vi "_Recursively Set BD Cluster Autosizing Property.vi"(8 "error in (no error)":errorcluster, 10 "type":T1(ring), 11 "SelList[]":refnum<vi>[](array[refnum])) -> (0 "error out":errorcluster, 3 "changed?":bool)   [LabVIEW 2017, in "Cluster AutoSizing.lvlib"]
uses:
  Cluster AutoSizing.lvlib
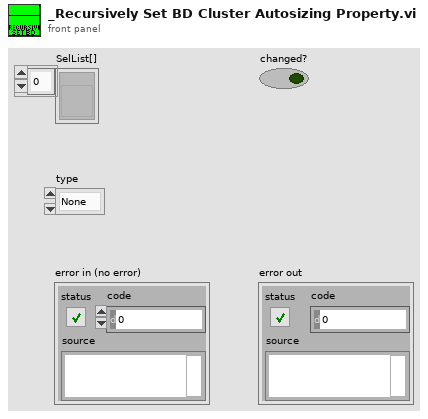
[diagram p1: front panel]
types:
  T1 = enum16{"None", "Size to Fit", "Arrange Horizontally", "Arrange Veritcally"}
  T2 = enum32{"None", "Size to Fit", "Arrange Horizontally", "Arrange Vertically"}
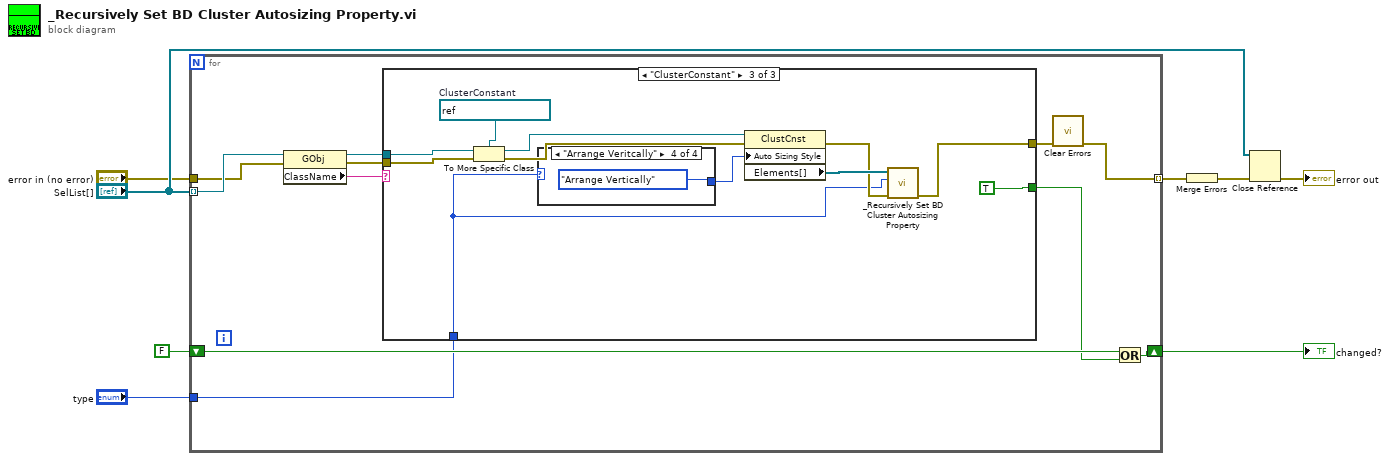
[diagram p0: block diagram]
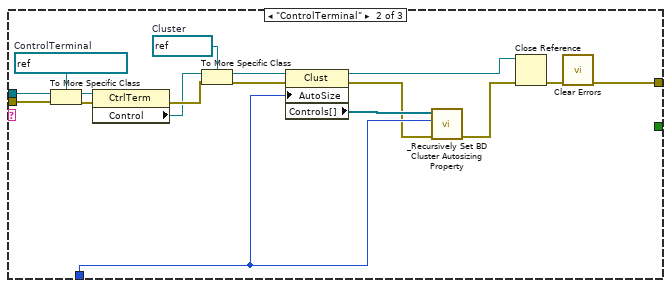
[diagram p3: hidden frame]
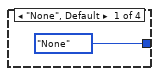
[diagram p4: hidden frame]
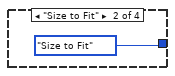
[diagram p5: hidden frame]
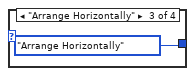
[diagram p6: hidden frame]
diagram:
  n1 = for {
    shift-right: [w18] -> w3
    shift-left: FALSE -> [w19]
    tunnel: "SelList[]" -> [w17] mode=indexing
    tunnel: "error in (no error)" -> [w12]
    tunnel: [w9] -> w4 mode=indexing
    tunnel: "type" -> [w16]
    n2 = property class="GObj"(reference=w17, error in=w12) -> (reference out=w14:refnum<vi>, error out=w13:errorcluster, "ClassName"=w11:string)
    n3 = case shown="\"ClusterConstant\"" w11 {
      tunnel: w16 -> [_ w23 w38]
      tunnel: [w20 w25 w39] -> w15
      tunnel: w14 -> [_ w30 w48]
      tunnel: w13 -> [w20 w29 w47]
      tunnel: [_ _ TRUE] -> w10
      frame Default {
      }
      frame "ControlTerminal" {
        w33 = refnum<vi> refnum  # Cluster
        w28 = refnum<vi> refnum  # ControlTerminal
        n4 = To More Specific Class(target class=w28, reference=w30, error in=w29) -> (specific class reference=w37:refnum<vi>, error out=w36:errorcluster)
        n5 = property class="CtrlTerm"(reference=w37, error in=w36) -> (error out=w32:errorcluster, "Control"=w27:refnum<vi>)  [unwired: 1 out]
        n6 = To More Specific Class(target class=w33, reference=w27, error in=w32) -> (specific class reference=w35:refnum<vi>, error out=w34:errorcluster)
        n7 = property class="Clust"(reference=w35, error in=w34, "AutoSize"=w23) -> (reference out=w31:refnum<vi>, error out=w22:errorcluster, "Controls[]"=w24:refnum<vi>[])
        n8 = call "_Recursively Set BD Cluster Autosizing Property.vi"("error in (no error)"=w22, "type"=w23, "SelList[]"=w24) -> ("error out"=w21:errorcluster)  [unwired: 7 in, 1 out]
        n9 = Close Reference(reference=w31, error in (no error)=w21) -> (error out=w26:errorcluster)
        n10 = call <vilib>:"Clear Errors.vi"("error in (no error)"=w26) -> ("error out"=w25:errorcluster)  [unwired: 5 in, 1 out]
      }
      frame "ClusterConstant" {
        w46 = refnum<vi> refnum  # ClusterConstant
        n11 = To More Specific Class(target class=w46, reference=w48, error in=w47) -> (specific class reference=w44:refnum<vi>, error out=w45:errorcluster)
        n12 = case shown="\"Arrange Veritcally\"" w38 {
          tunnel: [T2."None" ("Auto Sizing Style") T2."Size to Fit" ("Auto Sizing Style") T2."Arrange Horizontally" ("Auto Sizing Style") T2."Arrange Vertically" ("Auto Sizing Style")] -> w42
          frame "None", Default {
          }
          frame "Size to Fit" {
          }
          frame "Arrange Horizontally" {
          }
          frame "Arrange Veritcally" {
          }
        }
        n13 = property class="ClustCnst"(reference=w44, error in=w45, "Auto Sizing Style"=w42) -> (error out=w40:errorcluster, "Elements[]"=w41:refnum<vi>[])  [unwired: 1 out]
        n14 = call "_Recursively Set BD Cluster Autosizing Property.vi"("error in (no error)"=w40, "type"=w38, "SelList[]"=w41) -> ("error out"=w39:errorcluster)  [unwired: 7 in, 1 out]
      }
    }
    n15 = call <vilib>:"Clear Errors.vi"("error in (no error)"=w15) -> ("error out"=w9:errorcluster)  [unwired: 5 in, 1 out]
    n16 = Or(x=w19, y=w10) -> (x .or. y?=w18:bool)
  }
  "changed?" <- w3
  n17 = Merge Errors(w4) -> (w8:errorcluster)
  n18 = Close Reference(reference="SelList[]", error in (no error)=w8) -> (error out=→"error out":errorcluster)
